vi "Write messageID.vi"(8 "error in (no error)":errorcluster, 10 "messageID":u16, 11 "mqttCmd in":refnum<class "BaseMqttMsg.lvclass">) -> (0 "error out":errorcluster, 3 "mqttCmd out":refnum<class "BaseMqttMsg.lvclass">)   [LabVIEW 2020, in "BaseMqttMsg.lvclass"]
uses:
  BaseMqttMsg.lvclass
  BaseMqttMsg.lvclass/BaseMqttMsg.ctl
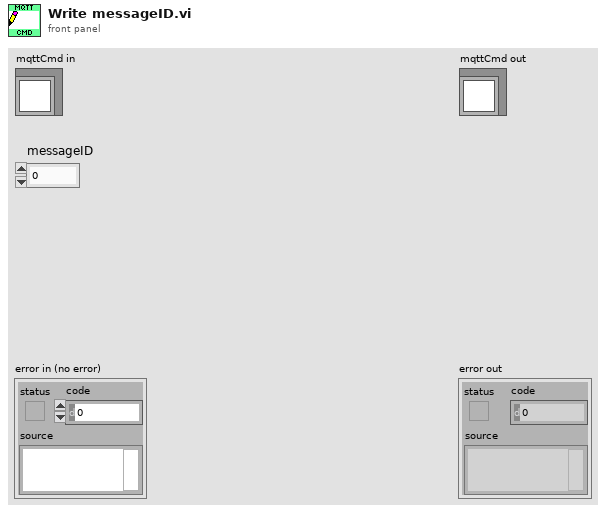
[diagram p1: front panel]
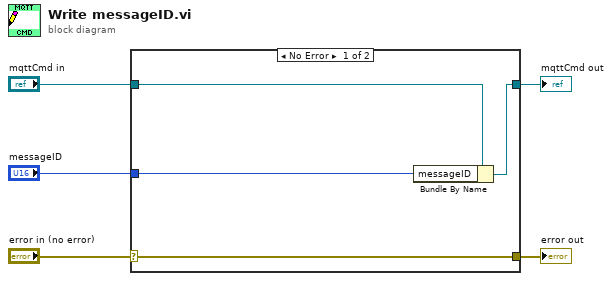
[diagram p0: block diagram]
diagram:
  n1 = case shown="No Error" "error in (no error)" {
    selector: "error in (no error)" -> [w9 w10]
    tunnel: [w9 w10] -> w4
    tunnel: [w7 w11] -> w2
    tunnel: "mqttCmd in" -> [w8 w11]
    tunnel: "messageID" -> [w6 _]
    frame No Error {
      n2 = Bundle By Name(cluster=w8, "messageID"=w6) -> (w7:refnum<class "BaseMqttMsg.lvclass">)
    }
    frame Error {
    }
  }
  "error out" <- w4
  "mqttCmd out" <- w2
